vi "Init.vi"(8 "error in (no error)":errorcluster, 11 "Device Class (All)":string) -> (0 "error out":errorcluster, 3 "Remote Systems out":refnum<class "Remote Systems.lvclass">)   [LabVIEW 2020, in "Remote Systems.lvclass"]
uses:
  Remote Systems.lvclass
  Remote Systems.lvclass/Remote Systems.ctl
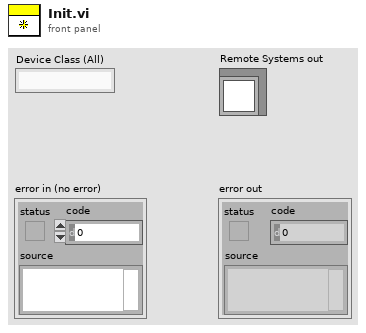
[diagram p1: front panel]
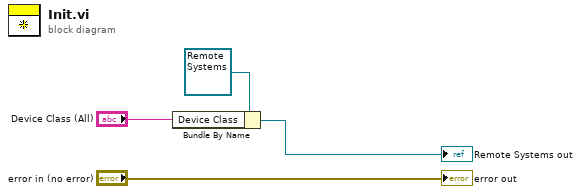
[diagram p0: block diagram]
diagram:
  n1 = Bundle By Name(cluster=refnum<class "Remote Systems.lvclass"> refnum ("Remote Systems in"), "Device Class"="Device Class (All)") -> (→"Remote Systems out":refnum<class "Remote Systems.lvclass">)
  "error out" <- "error in (no error)"
